vi "Sensor Scaling.vi"(8 "error in":errorcluster) -> (0 "error out":errorcluster, 3 "Output":cluster{"X":dbl[], "Y":dbl[], "Avg point":i16}[](array[cluster]))   [LabVIEW 2015]
uses:
  <vilib>/Analysis/NI_AALPro.lvlib
panel:
  in  "Avg Point":i16=1 min=1 max=500
  out "Offset":dbl format="%0.2f"
  out "Slope":dbl format="%0.2f"
  in  "Unit":string
  in  "Sensor":u16(ring) items=["Load Cell", "LVDT", "Clip Analog AI6", "Clip Analog AI7", "Clip Analog AI8", "Clip Analog A9", ""]
  in  "Next":bool
  in  "Input Values":dbl[](array[numeric])
  in  "New Calibration":dbl[](array[numeric])
  in  "Sensor Add":bool
  in  "Graph Plot":bool
  in  "Help Button":bool
  in  "Quit":bool
  in  "Save":bool
  out "XY Graph":T1(graph)
  out "error out 2":errorcluster
  out "Numeric":dbl
  out "Old Calibration":dbl[](array[numeric])
  # "Sensor Calibration"
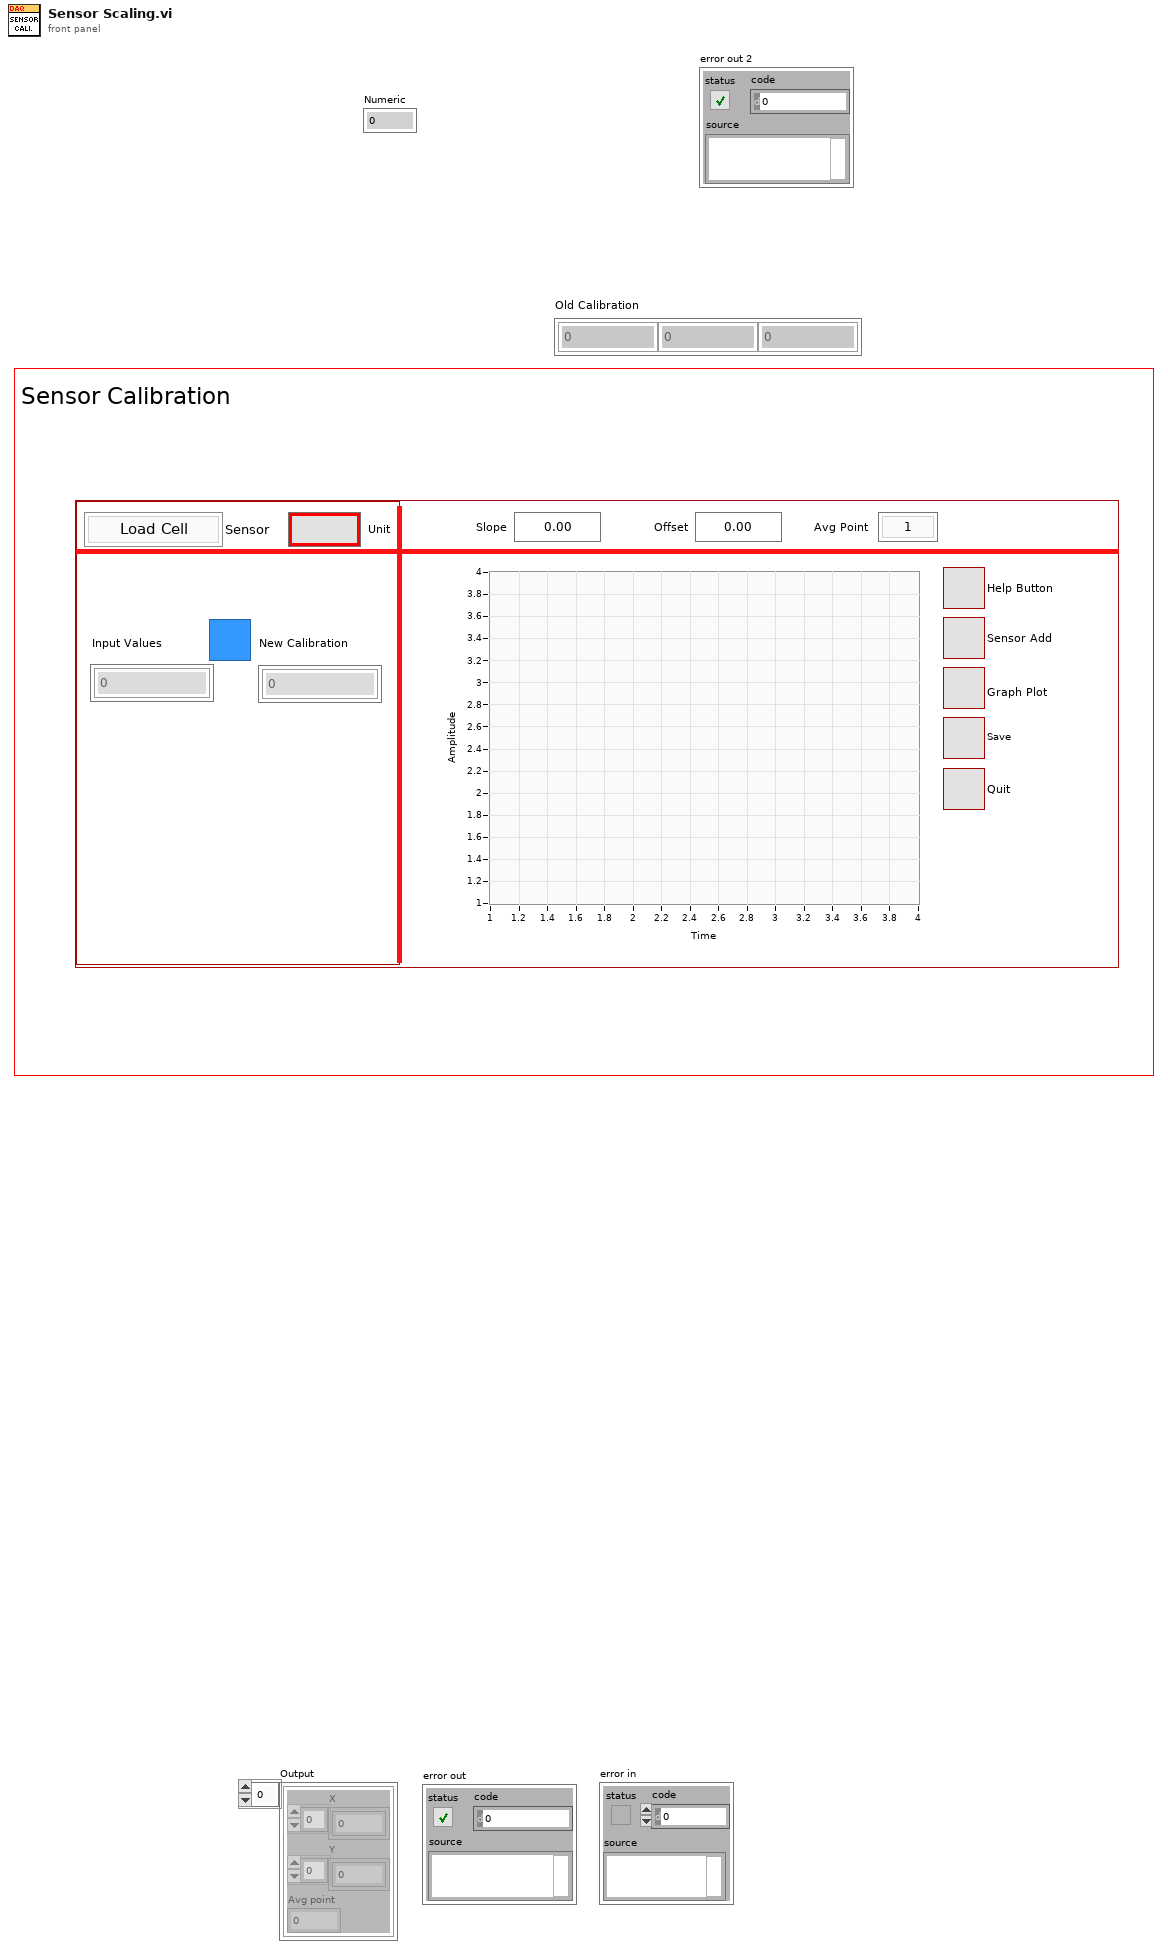
[diagram p1: front panel]
types:
  T1 = cluster{"Input Values":dbl[], "New Calibration":dbl[]}
  T2 = cluster{"XInput":dbl[], "Y New Value":dbl[], "Avg point":i16}[]
  T3 = cluster{"XInput":dbl[], "Y New Value":dbl[], "Avg point":i16}
  T4 = cluster{"Input Values":dbl[], "New Calibration":dbl[], "Sensor":u16}
  T5 = cluster{"Input Values":dbl[], "New Calibration":dbl[], "Avg point":i16}
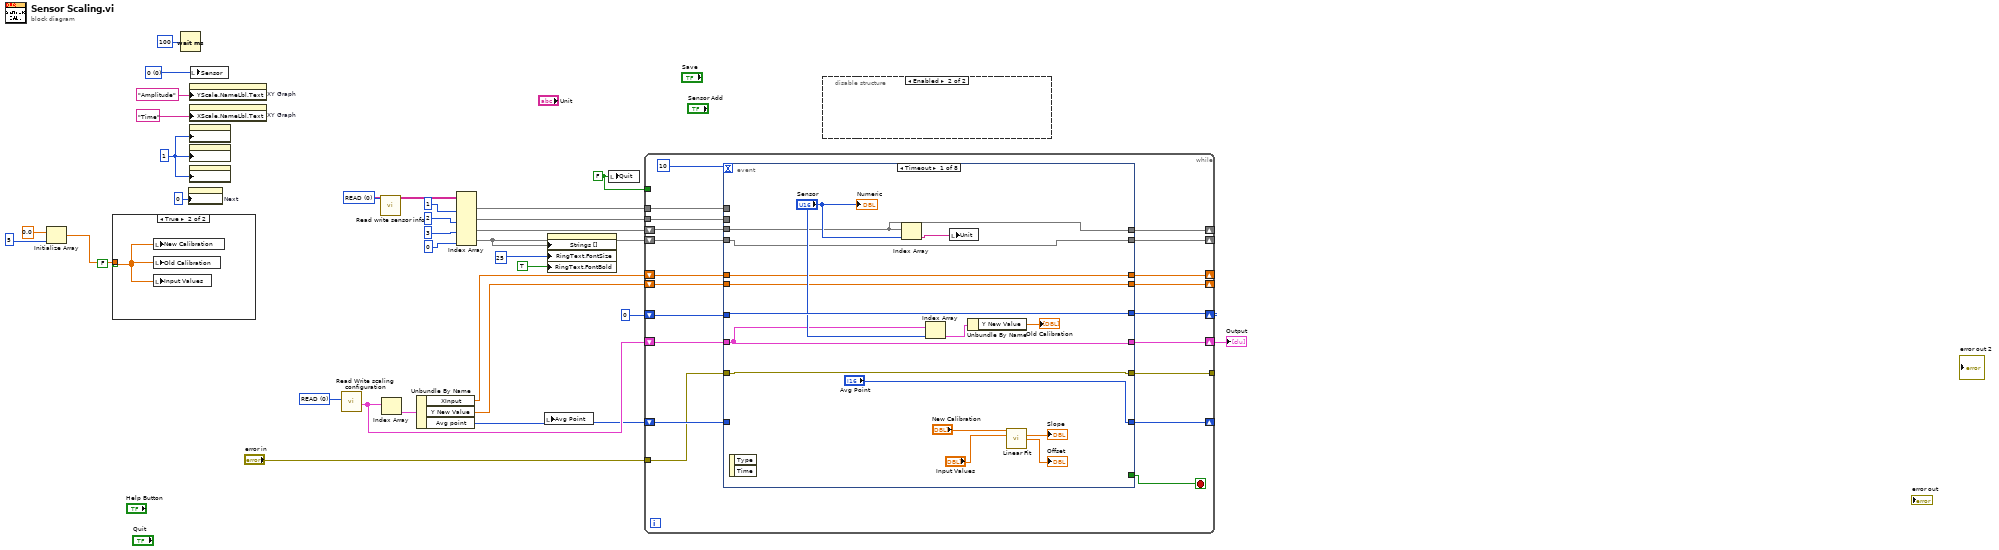
[diagram p0: block diagram]
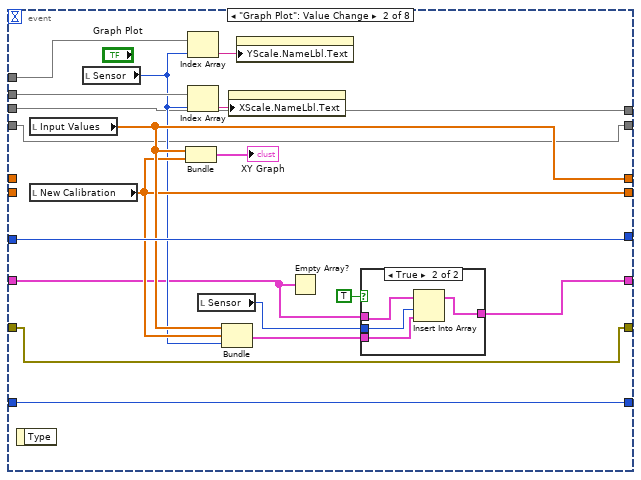
[diagram p4: hidden frame]
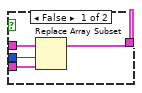
[diagram p5: hidden frame]
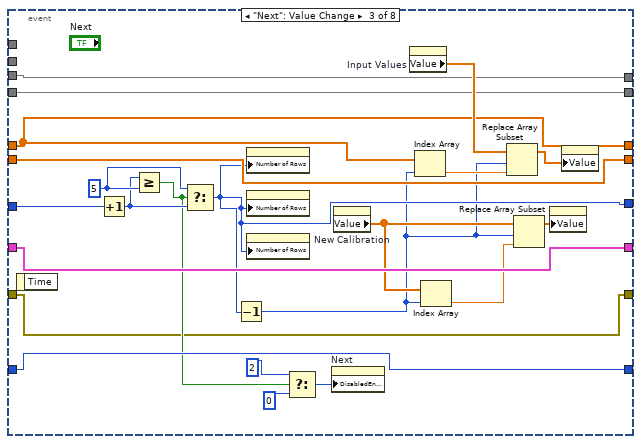
[diagram p6: hidden frame]
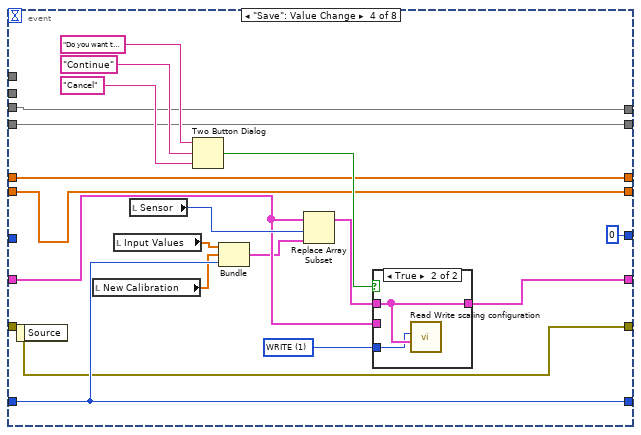
[diagram p7: hidden frame]
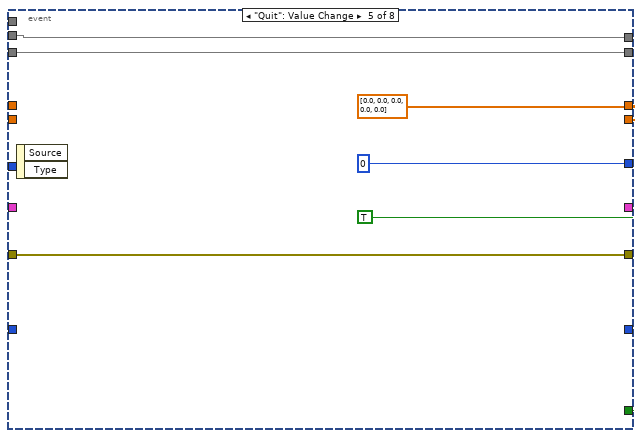
[diagram p9: hidden frame]
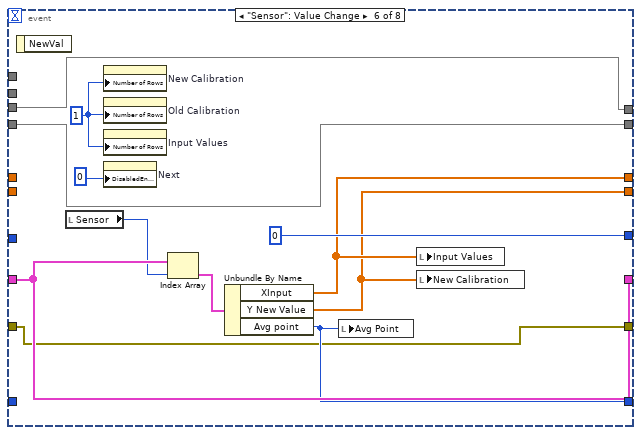
[diagram p10: hidden frame]
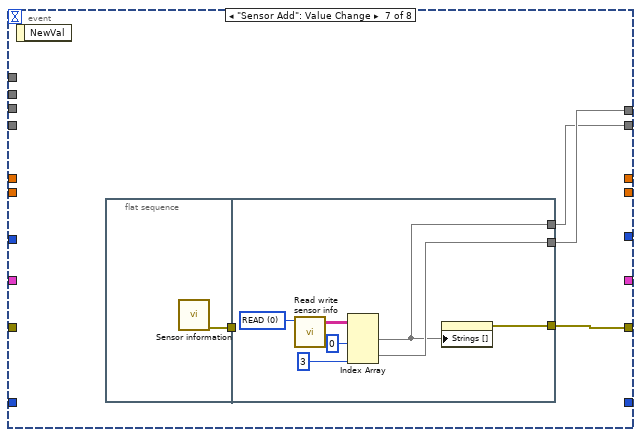
[diagram p11: hidden frame]
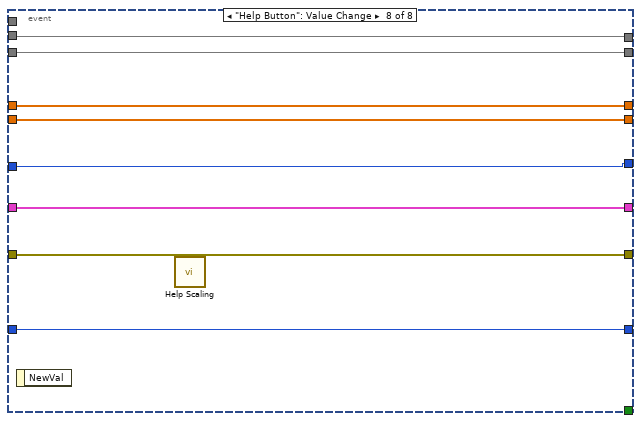
[diagram p12: hidden frame]
diagram:
  w5 = FALSE ("Quit")
  w15 = u16 0 items=["READ", "WRITE"] ("Read/Write")
  w21 = u16 0 items=["READ", "WRITE"] ("Read/Write")
  w11 = u32 1 ("Number of Rows")
  w29 = u16 0 items=["0", "1", "2", "3", "4", "5", "6", "7", "8", "9", "10", "11", "12", "13", "14", "15", "16", "17", "18", "19", "20", "21", "22", "23", "24", "25", "26", "27", "28", "29"] ("Ring")
  n1 = Initialize Array(0.0 ("element"), 5 ("dimension size")) -> (w2:dbl[])
  n2 = case shown="True" FALSE {
    tunnel: w2 -> [_ w33]
    frame False {
    }
    frame True {
      n3 = local write "New Calibration"(w33) -> ()
      n4 = local write "Old Calibration"(w33) -> ()
      n5 = local write "Input Values"(w33) -> ()
    }
  }
  n6 = Wait (ms)(milliseconds to wait=u32 100) -> ()  [unwired: 1 out]
  n7 = property on="Next" class="Bool"("DisabledEnum"=u16 0) -> ()  [unwired: 2 in, 2 out]
  n8 = property on="XY Graph" class="XYGraph (strict)"("YScale.NameLbl.Text"="Amplitude" ("Y Scale.Name Label.Text")) -> ()  [unwired: 2 in, 2 out]
  n9 = property on="XY Graph" class="XYGraph (strict)"("XScale.NameLbl.Text"="Time" ("X Scale.Unit Label.Text")) -> ()  [unwired: 2 in, 2 out]
  n10 = property on="Old Calibration" class="Arr (strict)"("Number of Rows"=w11) -> ()  [unwired: 2 in, 2 out]
  n11 = property on="Input Values" class="Arr (strict)"("Number of Rows"=w11) -> ()  [unwired: 2 in, 2 out]
  n12 = property on="New Calibration" class="Arr (strict)"("Number of Rows"=w11) -> ()  [unwired: 2 in, 2 out]
  n13 = local write "Sensor"(w29) -> ()
  n14 = call "Read Write scaling configuration.vi"("Read/Write"=w21) -> ("Output"=w19:T2)  [unwired: 4 in, 2 out]
  n15 = call "Read write sensor info.vi"("Read/Write"=w15) -> ("Table Control out"=w14:string[][])  [unwired: 9 in, 1 out]
  n16 = Index Array(array=w19) -> (element=w20:T3)  [unwired: 1 in]
  n17 = Unbundle By Name(w20) -> ("XInput"=w9:dbl[], "Y New Value"=w8:dbl[], "Avg point"=w18:i16)
  n18 = Index Array(array=w14, index (col) #1=1 ("disabled index (col)"), index (col) #2=2 ("index (row)"), index (col) #3=3 ("index (row)"), index (col) #4=0 ("index (row)")) -> (element #1=w26:string[], element #2=w25:string[], element #3=w7:string[], element #4=w6:string[])  [unwired: 4 in]
  n19 = local write "Avg Point"(w18) -> ()
  n20 = property on="Sensor" class="Ring (strict)"("Strings []"=w6, "RingText.FontSize"=u32 25 ("Ring Text.Font:Size"), "RingText.FontBold"=TRUE ("Ring Text.Font:Bold")) -> ()  [unwired: 2 in, 2 out]
  n21 = local write "Quit"(w5) -> ()
  n22 = while {
    shift-right: [w51] -> _
    shift-left: i8 0 -> [w52]
    shift-right: [w50] -> _
    shift-left: w8 -> [w49]
    tunnel: w26 -> [w47]
    tunnel: w25 -> [w46]
    shift-right: [w45] -> _
    shift-left: w9 -> [w44]
    shift-right: [w42] -> w17
    shift-left: w19 -> [w43]
    shift-right: [w41] -> _
    shift-left: w18 -> [w40]
    tunnel: [w38] -> _
    tunnel: "error in" -> [w35]
    shift-right: [w37] -> _
    shift-left: w7 -> [w36]
    shift-right: [w34] -> _
    shift-left: w6 -> [w39]
    tunnel: w5 -> [_]
    stop <- w48 stop-if-true
    n23 = event shown="[0] Timeout" {
      selector: _ -> [_ _ _ _ _ _ _ _]
      dyn-events: _ -> [_ _ _ _ _ _ _ _]
      timeout: 10 -> [_ _ _ _ _ _ _ _]
      tunnel: [_ _ _ _ TRUE _ _ _] -> w48
      tunnel: w52 -> [w69 w83 w117 _ _ _ _ w172]
      tunnel: [w69 w83 w107 i8 0 i8 0 i8 0 ("y") _ w172] -> w51
      tunnel: [w63 w77 w113 w125 w143 w149 _ w175] -> w50
      tunnel: w49 -> [w63 _ w113 w125 _ _ _ w175]
      tunnel: w47 -> [_ w87 _ _ _ _ _ _]
      tunnel: w46 -> [_ w86 _ _ _ _ _ _]
      tunnel: w36 -> [w57 w72 w98 w123 w142 w148 _ w177]
      tunnel: [w64 w78 w110 w126 w143 w150 _ w176] -> w45
      tunnel: w44 -> [w64 _ w110 w126 _ _ _ w176]
      tunnel: w43 -> [w65 w74 w114 w128 _ w156 _ w174]
      tunnel: [w65 w75 w114 w131 _ w156 _ w174] -> w42
      tunnel: ["Avg Point" w82 w106 w129 _ w153 _ w173] -> w41
      tunnel: w40 -> [_ w82 w106 w129 _ _ _ w173]
      tunnel: w39 -> [w55 w70 w96 w121 w140 w146 _ w170]
      tunnel: [w56 w71 w97 w122 w141 w147 w160 w171] -> w38
      tunnel: [w57 w72 w98 w123 w142 w148 w159 w177] -> w37
      tunnel: w35 -> [w56 w71 w97 w122 w141 w147 _ w171]
      tunnel: [w55 w70 w96 w121 w140 w146 w158 w170] -> w34
      event Timeout {
        n24 = event-data() -> ()  [unwired: 3 out]
        n25 = Index Array(array=w57, index="Sensor") -> (element=w54:string)
        n26 = Index Array(array=w65, index="Sensor") -> (element=w67:T3)
        n27 = local write "Unit"(w54) -> ()
        n28 = Unbundle By Name(w67) -> ("Y New Value"=→"Old Calibration":dbl[])
        n29 = call <vilib>:"Linear Fit.vi"("Y"="New Calibration", "X"="Input Values") -> ("slope"=→"Slope":dbl, "intercept"=→"Offset":dbl)  [unwired: 9 in, 3 out]
        "Numeric" <- "Sensor"
      }
      event "Graph Plot": Value Change {
        n30 = event-data() -> ()  [unwired: 2 out]
        n31 = local read "Input Values"() -> (w78:dbl[])
        n32 = local read "New Calibration"() -> (w77:dbl[])
        n33 = local read "Sensor"() -> (w76:u16)
        n34 = Bundle("Input Values"=w78, "New Calibration"=w77) -> (→"XY Graph":T1)  [unwired: 1 in]
        n35 = Index Array(array=w87, index=w76) -> (element=w85:string)
        n36 = Index Array(array=w86, index=w76) -> (element=w84:string)
        n37 = local read "Sensor"() -> (w79:u16)
        n38 = Bundle("Input Values"=w78, "New Calibration"=w77, "Sensor"=w76) -> (w80:T4)  [unwired: 1 in]
        n39 = property on="XY Graph" class="XYGraph (strict)"("XScale.NameLbl.Text"=w84) -> ()  [unwired: 2 in, 2 out]
        n40 = property on="XY Graph" class="XYGraph (strict)"("YScale.NameLbl.Text"=w85) -> ()  [unwired: 2 in, 2 out]
        n41 = Empty Array?(array=w74) -> ()  [unwired: 1 out]
        n42 = case shown="True" TRUE {
          tunnel: w80 -> [w91 w93]
          tunnel: w79 -> [w90 w95]
          tunnel: w74 -> [w89 w94]
          tunnel: [w88 w92] -> w75
          frame False {
            n43 = Replace Array Subset(array=w89, new element=w91, index=w90) -> (w88:T2)
          }
          frame True {
            n44 = Insert Into Array(array=w94, index=w95, new element=w93) -> (w92:T2)
          }
        }
      }
      event "Next": Value Change {
        w116 = i8 5 ("y")
        n45 = event-data() -> ()  [unwired: 2 out]
        n46 = Increment(x=w117) -> (x+1=w115:i8)
        n47 = Greater Or Equal?(x=w115, y=w116) -> (x >= y?=w105:bool)
        n48 = Select(t=w116, s=w105, f=w115) -> (s? t:f=w107:i8)
        n49 = Decrement(x=w107) -> (x-1=w100:i8)
        n50 = property on="New Calibration" class="Arr (strict)"("Number of Rows"=w107) -> ()  [unwired: 2 in, 2 out]
        n51 = property on="Old Calibration" class="Arr (strict)"("Number of Rows"=w107) -> ()  [unwired: 2 in, 2 out]
        n52 = property on="Input Values" class="Arr (strict)"("Number of Rows"=w107) -> ()  [unwired: 2 in, 2 out]
        n53 = Select(t=2, s=w105, f=0) -> (s? t:f=w102:i32)
        n54 = property on="Next" class="Bool"("DisabledEnum"=w102) -> ()  [unwired: 2 in, 2 out]
        n55 = property on="New Calibration" class="Arr (strict)"() -> ("Value"=w101:dbl[])  [unwired: 2 in, 2 out]
        n56 = property on="Input Values" class="Arr (strict)"() -> ("Value"=w111:dbl[])  [unwired: 2 in, 2 out]
        n57 = Index Array(array=w110, index=w100) -> (element=w109:dbl)
        n58 = Index Array(array=w101, index=w100) -> (element=w99:dbl)
        n59 = Replace Array Subset(array=w111, new element=w109, index=w100) -> (w112:dbl[])
        n60 = Replace Array Subset(array=w101, new element=w99, index=w100) -> (w108:dbl[])
        n61 = property on="New Calibration" class="Arr (strict)"("Value"=w108) -> ()  [unwired: 2 in, 2 out]
        n62 = property on="Input Values" class="Arr (strict)"("Value"=w112) -> ()  [unwired: 2 in, 2 out]
      }
      event "Save": Value Change {
        w124 = u16 1 items=["READ", "WRITE"] ("Read/Write")
        n63 = event-data() -> ()  [unwired: 2 out]
        n64 = local read "New Calibration"() -> (w119:dbl[])
        n65 = local read "Input Values"() -> (w120:dbl[])
        n66 = local read "Sensor"() -> (w130:u16)
        n67 = Two Button Dialog(message="Do you want to save new calibration value?", 1:"Cancel" ("T button name (\"OK\")"), 2:"Continue" ("F button name (\"Cancel\")")) -> (T button?=w132:bool)
        n68 = Bundle("Input Values"=w120, "New Calibration"=w119, "Avg point"=w129) -> (w118:T5)  [unwired: 1 in]
        n69 = Replace Array Subset(array=w128, new element=w118, index=w130) -> (w127:T2)
        n70 = case shown="True" w132 {
          tunnel: w127 -> [_ w139]
          tunnel: [w137 w139] -> w131
          tunnel: w128 -> [w137 _]
          tunnel: w124 -> [_ w138]
          frame False {
          }
          frame True {
            n71 = call "Read Write scaling configuration.vi"("Input"=w139, "Read/Write"=w138) -> ()  [unwired: 3 in, 3 out]
          }
        }
      }
      event "Quit": Value Change {
        w143 = dbl[] [0.0, 0.0, 0.0, 0.0, 0.0]
        n72 = event-data() -> ()  [unwired: 3 out]
      }
      event "Sensor": Value Change {
        w151 = u32 1 ("Number of Rows")
        n73 = event-data() -> ()  [unwired: 2 out]
        n74 = local read "Sensor"() -> (w154:u16)
        n75 = property on="New Calibration" class="Arr (strict)"("Number of Rows"=w151) -> ()  [unwired: 2 in, 2 out]
        n76 = property on="Old Calibration" class="Arr (strict)"("Number of Rows"=w151) -> ()  [unwired: 2 in, 2 out]
        n77 = property on="Input Values" class="Arr (strict)"("Number of Rows"=w151) -> ()  [unwired: 2 in, 2 out]
        n78 = property on="Next" class="Bool"("DisabledEnum"=0) -> ()  [unwired: 2 in, 2 out]
        n79 = Index Array(array=w156, index=w154) -> (element=w157:T3)
        n80 = Unbundle By Name(w157) -> ("XInput"=w150:dbl[], "Y New Value"=w149:dbl[], "Avg point"=w153:i16)
        n81 = local write "Avg Point"(w153) -> ()
        n82 = local write "Input Values"(w150) -> ()
        n83 = local write "New Calibration"(w149) -> ()
      }
      event "Sensor Add": Value Change {
        n84 = event-data() -> ()  [unwired: 2 out]
        n85 = flat-sequence {
          tunnel: [w162] -> w161
          tunnel: w161 -> [_]
          tunnel: [w166] -> w160
          tunnel: [w164] -> w159
          tunnel: [w163] -> w158
          frame #0 {
            n86 = call "Sensor information.vi"() -> ("error in (no error) 2"=w162:errorcluster)  [unwired: 11 in]
          }
          frame #1 {
            w169 = u16 0 items=["READ", "WRITE"] ("Read/Write")
            n87 = call "Read write sensor info.vi"("Read/Write"=w169) -> ("Table Control out"=w168:string[][])  [unwired: 9 in, 1 out]
            n88 = Index Array(array=w168, index (col) #1=0 ("disabled index (col)"), index (col) #2=3 ("index (col)")) -> (element #1=w163:string[], element #2=w164:string[])  [unwired: 2 in]
            n89 = property on="Sensor" class="Ring (strict)"("Strings []"=w163) -> (error out=w166:errorcluster)  [unwired: 2 in, 1 out]
          }
        }
      }
      event "Help Button": Value Change {
        n90 = event-data() -> ()  [unwired: 2 out]
        n91 = call "Help Scaling.vi"() -> ()  [unwired: 12 in]
      }
    }
  }
  "Output" <- w17
  n92 = disable-structure shown="Enabled" {
    frame Disabled {
    }
    frame Enabled {
    }
  }
